vi "EXA_acceptCommand_exitControl.vi"(8 "error in (no error)":errorcluster, 11 "command_exitControl_Ctl":T1) -> (0 "error out":errorcluster, 2 "function return":i32, 3 "command_exitControl_Ctl out":T1)   [LabVIEW 2016, in "SALLV_EXA.lvlib"]
doc: "int EXA_shm_acceptCommand_exitControlLV(EXA_command_exitControlLV *command_exitControl_Ctl );"
uses:
  SALLV_EXA.lvlib
  DataTypes/command_exitControl.ctl
  SALLV_EXA.so
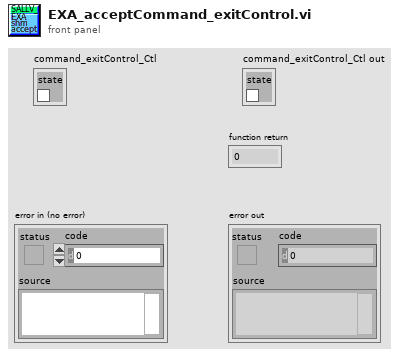
[diagram p1: front panel]
types:
  T1 = typedef "SALLV_EXA.lvlib/command_exitControl.ctl" = cluster{"state":bool}
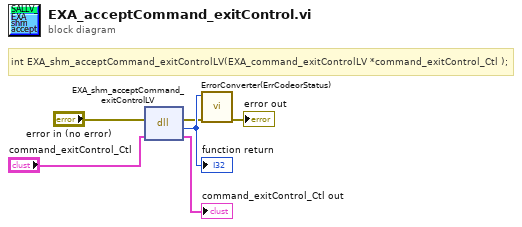
[diagram p0: block diagram]
diagram:
  # "int EXA_shm_acceptCommand_exitControlLV(EXA_command_exitControlLV *command_exitControl_Ctl );"
  n1 = dll-call lib="home/andres/Desktop/EXA_SAL_LV/SALLV_EXA.*" fn="EXA_shm_acceptCommand_exitControlLV"(error in="error in (no error)", "command_exitControl_Ctl"="command_exitControl_Ctl") -> (error out=w2:errorcluster, w6:i32, "command_exitControl_Ctl"=→"command_exitControl_Ctl out":T1)  [unwired: 2 in, 1 out]
  "function return" <- w6
  n2 = call "ErrorConverter(ErrCodeorStatus).vi"("error in (no error)"=w2, "error code"=w6) -> ("error out"=→"error out":errorcluster)  [unwired: 9 in]
